vi "PH_Sequencer.PC _Head_in_Use.vi"(0 "VI in":refnum<vi>, 2 "Service Name in Use":string, 3 "in Use?":bool, 4 "no link?":bool, 5 "error in (no error)":errorcluster) -> (14 "VI out":refnum<vi>, 19 "error out":errorcluster)   [LabVIEW 2014, in "PH_Sequencer.lvlib"]
doc: "This VI stores information at own attributes and forces some action."
uses:
  PH_Sequencer.lvlib
  PH_PP_Common/PH_PP_Common.PUs.ctl
  PH_BeamlineInformation/PH_BeamlineInformation.lvlib
  PH_PP_Common/PH_PP_Common.lvlib
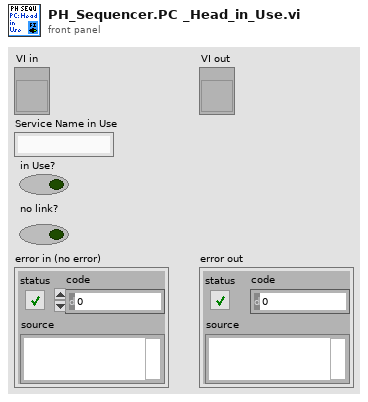
[diagram p1: front panel]
types:
  T1 = typedef "PH_PP_Common.lvlib/PH_PP_Common.PUs.ctl" = enum16{"no Info", "PA-19mm-1", "PA-19mm-2", "PA-45mm-PILC", "PA-45mm-MAIN", "MA-PU-1", "MA-PU-2", "MA-PU-3", "MA-PU-4", "MA-PU-5", "MA-PU-6", "MA-FR", "MA-PILC", "PA-45mm-DP"}
  T2 = typedef "PH_BeamlineInformation.lvlib/PH_BeamlineInformation.i attribute.ctl" = cluster{"BL GUI Elements of Services":cluster{"Service Name":string, "GUI Elements":refnum<vi>[], "Status":i32}[], "Powermeters":T3, "Efficiency":T4, "Heads":T5[]}
  T3 = typedef "PH_BeamlineInformation.lvlib/PH_BeamlineInformation.Powermeter.ctl" = cluster{"ns FE":cluster{"GUI Ref":refnum<vi>, "Value":dbl}, "fs FE":cluster{"GUI Ref":refnum<vi>, "Value":dbl}, "PA":cluster{"GUI Ref":refnum<vi>, "Value":dbl}, "MA":cluster{"GUI Ref":refnum<vi>, "Value":dbl}, "Z6 green":cluster{"GUI Ref":refnum<vi>, "Value":dbl}, "Z6 IR":cluster{"GUI Ref":refnum<vi>, "Value":dbl}, "Z6 COS":cluster{"GUI Ref":refnum<vi>, "Value":dbl}}
  T4 = typedef "PH_BeamlineInformation.lvlib/PH_BeamlineInformation.Efficiency.ctl" = cluster{"PA Gain":cluster{"GUI Ref":refnum<vi>, "Value":dbl}, "MA Gain":cluster{"GUI Ref":refnum<vi>, "Value":dbl}, "Z6 green Conversion":cluster{"GUI Ref":refnum<vi>, "Value":dbl}, "Z6 Comp Losses":cluster{"GUI Ref":refnum<vi>, "Value":dbl}}
  T5 = typedef "PH_BeamlineInformation.lvlib/PH_BeamlineInformation.Head.ctl" = cluster{"PowerUnit":T1, "in use":cluster{"Value":bool, "GUI Ref":refnum<vi>, "linked":bool}, "voltage":cluster{"Value":dbl, "GUI Ref":refnum<vi>, "linked":bool}}
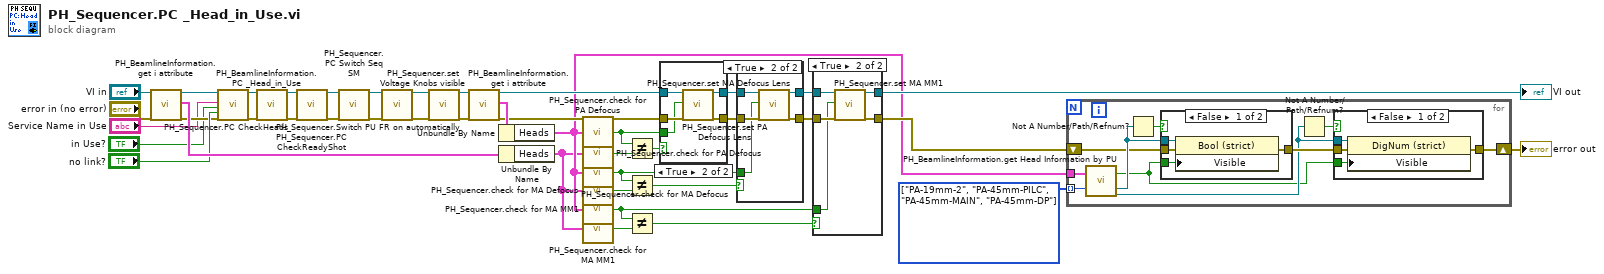
[diagram p0: block diagram]
diagram:
  w16 = T1[] [enum."PA-19mm-2", enum."PA-45mm-PILC", enum."PA-45mm-MAIN", enum."PA-45mm-DP"] items=["no Info", "PA-19mm-1", "PA-19mm-2", "PA-45mm-PILC", "PA-45mm-MAIN", "MA-PU-1", "MA-PU-2", "MA-PU-3", "MA-PU-4", "MA-PU-5", "MA-PU-6", "MA-FR", "MA-PILC", "PA-45mm-DP"]
  n1 = call "PH_BeamlineInformation.get i attribute.vi"("i ref in"="VI in", "error in (no error)"="error in (no error)") -> ("i ref out"=w37:refnum<vi>, "i attribute"=w40:T2, "error out"=w35:errorcluster)  [unwired: 15 in]
  n2 = call "PH_BeamlineInformation.PC _Head_in_Use.vi"("i ref in"=w37, "In Use Service Name"="Service Name in Use", "In Use?"="in Use?", "no link?"="no link?", "error in (no error)"=w35) -> ("i ref out"=w32:refnum<vi>, "error out"=w31:errorcluster)  [unwired: 13 in]
  n3 = call "PH_Sequencer.PC CheckHeads.vi"("i ref in"=w32, "error in (no error)"=w31) -> ("i ref out"=w42:refnum<vi>, "error out"=w41:errorcluster)  [unwired: 16 in]
  n4 = call "PH_Sequencer.PC CheckReadyShot.vi"("i ref in"=w42, "error in (no error)"=w41) -> ("i ref out"=w30:refnum<vi>, "error out"=w29:errorcluster)  [unwired: 16 in]
  n5 = call "PH_Sequencer.PC Switch Seq SM.vi"("i ref in"=w30, "error IO"=w29) -> ("i ref out"=w21:refnum<vi>, "error out"=w23:errorcluster)  [unwired: 16 in]
  n6 = call "PH_Sequencer.set Voltage Knobs visible.vi"("VI in"=w21, "error in (no error)"=w23) -> ("VI out"=w20:refnum<vi>, "error out"=w22:errorcluster)  [unwired: 16 in]
  n7 = call "PH_Sequencer.Switch PU FR on automatically.vi"("i ref in"=w20, "error in"=w22) -> ("i ref out"=w24:refnum<vi>, "error out"=w25:errorcluster)  [unwired: 16 in]
  n8 = call "PH_BeamlineInformation.get i attribute.vi"("i ref in"=w24, "error in (no error)"=w25) -> ("i ref out"=w27:refnum<vi>, "i attribute"=w28:T2, "error out"=w26:errorcluster)  [unwired: 15 in]
  n9 = Unbundle By Name(w28) -> ("Heads"=w7:T5[])
  n10 = Unbundle By Name(w40) -> ("Heads"=w6:T5[])
  n11 = call "PH_Sequencer.check for PA Defocus.vi"("Heads"=w7) -> ("PA Defocus must be set?"=w3:bool)
  n12 = call "PH_Sequencer.check for PA Defocus.vi"("Heads"=w6) -> ("PA Defocus must be set?"=w15:bool)
  n13 = call "PH_Sequencer.check for MA Defocus.vi"("Heads"=w7) -> ("MA Defocus must be set?"=w2:bool)
  n14 = call "PH_Sequencer.check for MA Defocus.vi"("Heads"=w6) -> ("MA Defocus must be set?"=w9:bool)
  n15 = call "PH_Sequencer.check for MA MM1.vi"("Heads"=w7) -> ("MA MM1 must be set?"=w1:bool)
  n16 = call "PH_Sequencer.check for MA MM1.vi"("Heads"=w6) -> ("MA MM1 must be set?"=w5:bool)
  n17 = Not Equal?(x=w3, y=w15) -> (x != y?=w14:bool)
  n18 = Not Equal?(x=w2, y=w9) -> (x != y?=w8:bool)
  n19 = Not Equal?(x=w1, y=w5) -> (x != y?=w4:bool)
  n20 = case shown="True" w14 {
    tunnel: [w44 w49] -> w13
    tunnel: w27 -> [w44 w48]
    tunnel: [w43 w47] -> w11
    tunnel: w26 -> [w43 w46]
    tunnel: w3 -> [_ w45]
    frame False {
    }
    frame True {
      n21 = call "PH_Sequencer.set PA Defocus Lens.vi"("i ref in"=w48, "Shotposition?"=w45, "error in"=w46) -> ("i ref out"=w49:refnum<vi>, "error out"=w47:errorcluster)  [unwired: 15 in]
    }
  }
  n22 = case shown="True" w8 {
    tunnel: [w51 w56] -> w12
    tunnel: w13 -> [w51 w55]
    tunnel: [w50 w54] -> w10
    tunnel: w11 -> [w50 w53]
    tunnel: w2 -> [_ w52]
    frame False {
    }
    frame True {
      n23 = call "PH_Sequencer.set MA Defocus Lens.vi"("i ref in"=w55, "Shotposition?"=w52, "error in"=w53) -> ("i ref out"=w56:refnum<vi>, "error out"=w54:errorcluster)  [unwired: 15 in]
    }
  }
  n24 = case shown="True" w4 {
    tunnel: w10 -> [w57 w60]
    tunnel: [w57 w62] -> w17
    tunnel: w12 -> [w58 w61]
    tunnel: [w58 w63] -> w18
    tunnel: w1 -> [_ w59]
    frame False {
    }
    frame True {
      n25 = call "PH_Sequencer.set MA MM1.vi"("i ref in"=w61, "High Energy Position?"=w59, "error in"=w60) -> ("i ref out"=w63:refnum<vi>, "error out"=w62:errorcluster)  [unwired: 15 in]
    }
  }
  "VI out" <- w18
  n26 = for {
    tunnel: w7 -> [w73]
    tunnel: w16 -> [w68] mode=indexing
    shift-right: [w66] -> w19
    shift-left: w17 -> [w65]
    n27 = call "PH_BeamlineInformation.get Head Information by PU.vi"("Heads"=w73, "Power Unit"=w68) -> ("In Use linked?"=w64:bool, "In Use GUI Ref"=w67:refnum<vi>, "Voltage GUI Ref"=w69:refnum<vi>)  [unwired: 12 in, 3 out]
    n28 = Not A Number/Path/Refnum?(number/path/refnum=w67) -> (NaN/Path/Refnum?=w72:bool)
    n29 = case shown="False" w72 {
      tunnel: w65 -> [w82 w83]
      tunnel: [w81 w83] -> w70
      tunnel: w67 -> [w80 _]
      tunnel: w64 -> [w79 _]
      frame False {
        n30 = property class="Bool (strict)"(reference=w80, error in=w82, "Visible"=w79) -> (error out=w81:errorcluster)  [unwired: 1 out]
      }
      frame True {
      }
    }
    n31 = Not A Number/Path/Refnum?(number/path/refnum=w69) -> (NaN/Path/Refnum?=w71:bool)
    n32 = case shown="False" w71 {
      tunnel: w70 -> [w77 w78]
      tunnel: [w76 w78] -> w66
      tunnel: w69 -> [w75 _]
      tunnel: w64 -> [w74 _]
      frame False {
        n33 = property class="DigNum (strict)"(reference=w75, error in=w77, "Visible"=w74) -> (error out=w76:errorcluster)  [unwired: 1 out]
      }
      frame True {
      }
    }
  }
  "error out" <- w19
